vi "Teleop.vi"(10 "Match Info":T2={"Autonomous Elapsed Seconds"=0.0, "TeleOp Elapsed Seconds"=0.0, "Disabled Elapsed Seconds"=0.0, "Visited Autonomous"=FALSE, "Visited TeleOp"=FALSE, "Visited Disabled"=FALSE, "Autonomous Settings"={"Autonomous Style"=enum."Independent", "VI Refnum"=refnum}}, 11 "Call Context":T3) -> ()   [LabVIEW 2020]
doc: "This VI is called for each TeleOp packet received from the DS where the robot is not disabled. It is often used to read from the joysticks and update I/O or to update setpoints for timed control loops. It should complete and return within 20 milliseconds or it may miss DS packets."
uses:
  <vilib>/Rock Robotics/WPI/DriverStation/WPI_DriverStationDerivedRobotMode.ctl
  <vilib>/Rock Robotics/WPI/DriverStation/WPI_DriverStationMatch Info.ctl
  <vilib>/Rock Robotics/WPI/ThirdParty/Phoenix-LabVIEW/Motor Controller/Controls/CTRE_Phoenix_MotorControl_ControlMode.ctl
  <vilib>/Rock Robotics/WPI/ThirdParty/Phoenix-LabVIEW/CANCoder/Get/CTRE_Phoenix_CANcoder_GetSensorData.vi
  <vilib>/Rock Robotics/WPI/ThirdParty/Phoenix-LabVIEW/Pigeon IMU/CTRE_PigeonIMU_GetYPR.vi
panel:
  in  "FR PID gains":T1={"proportional gain (Kc)"=0.01, "integral time (Ti, min)"=0.0, "derivative time (Td, min)"=0.0} {"derivative time (Td, min)" format="%.3f"; "integral time (Ti, min)" format="%.3f"; "proportional gain (Kc)" format="%.6f"}
  in  "FL PID gains":T1={"proportional gain (Kc)"=0.01, "integral time (Ti, min)"=0.0, "derivative time (Td, min)"=0.0} {"derivative time (Td, min)" format="%.3f"; "integral time (Ti, min)" format="%.3f"; "proportional gain (Kc)" format="%.6f"}
  in  "BR PID gains":T1={"proportional gain (Kc)"=0.01, "integral time (Ti, min)"=0.0, "derivative time (Td, min)"=0.0} {"derivative time (Td, min)" format="%.3f"; "integral time (Ti, min)" format="%.3f"; "proportional gain (Kc)" format="%.6f"}
  in  "BL PID gains":T1={"proportional gain (Kc)"=0.01, "integral time (Ti, min)"=0.0, "derivative time (Td, min)"=0.0} {"derivative time (Td, min)" format="%.3f"; "integral time (Ti, min)" format="%.3f"; "proportional gain (Kc)" format="%.6f"}
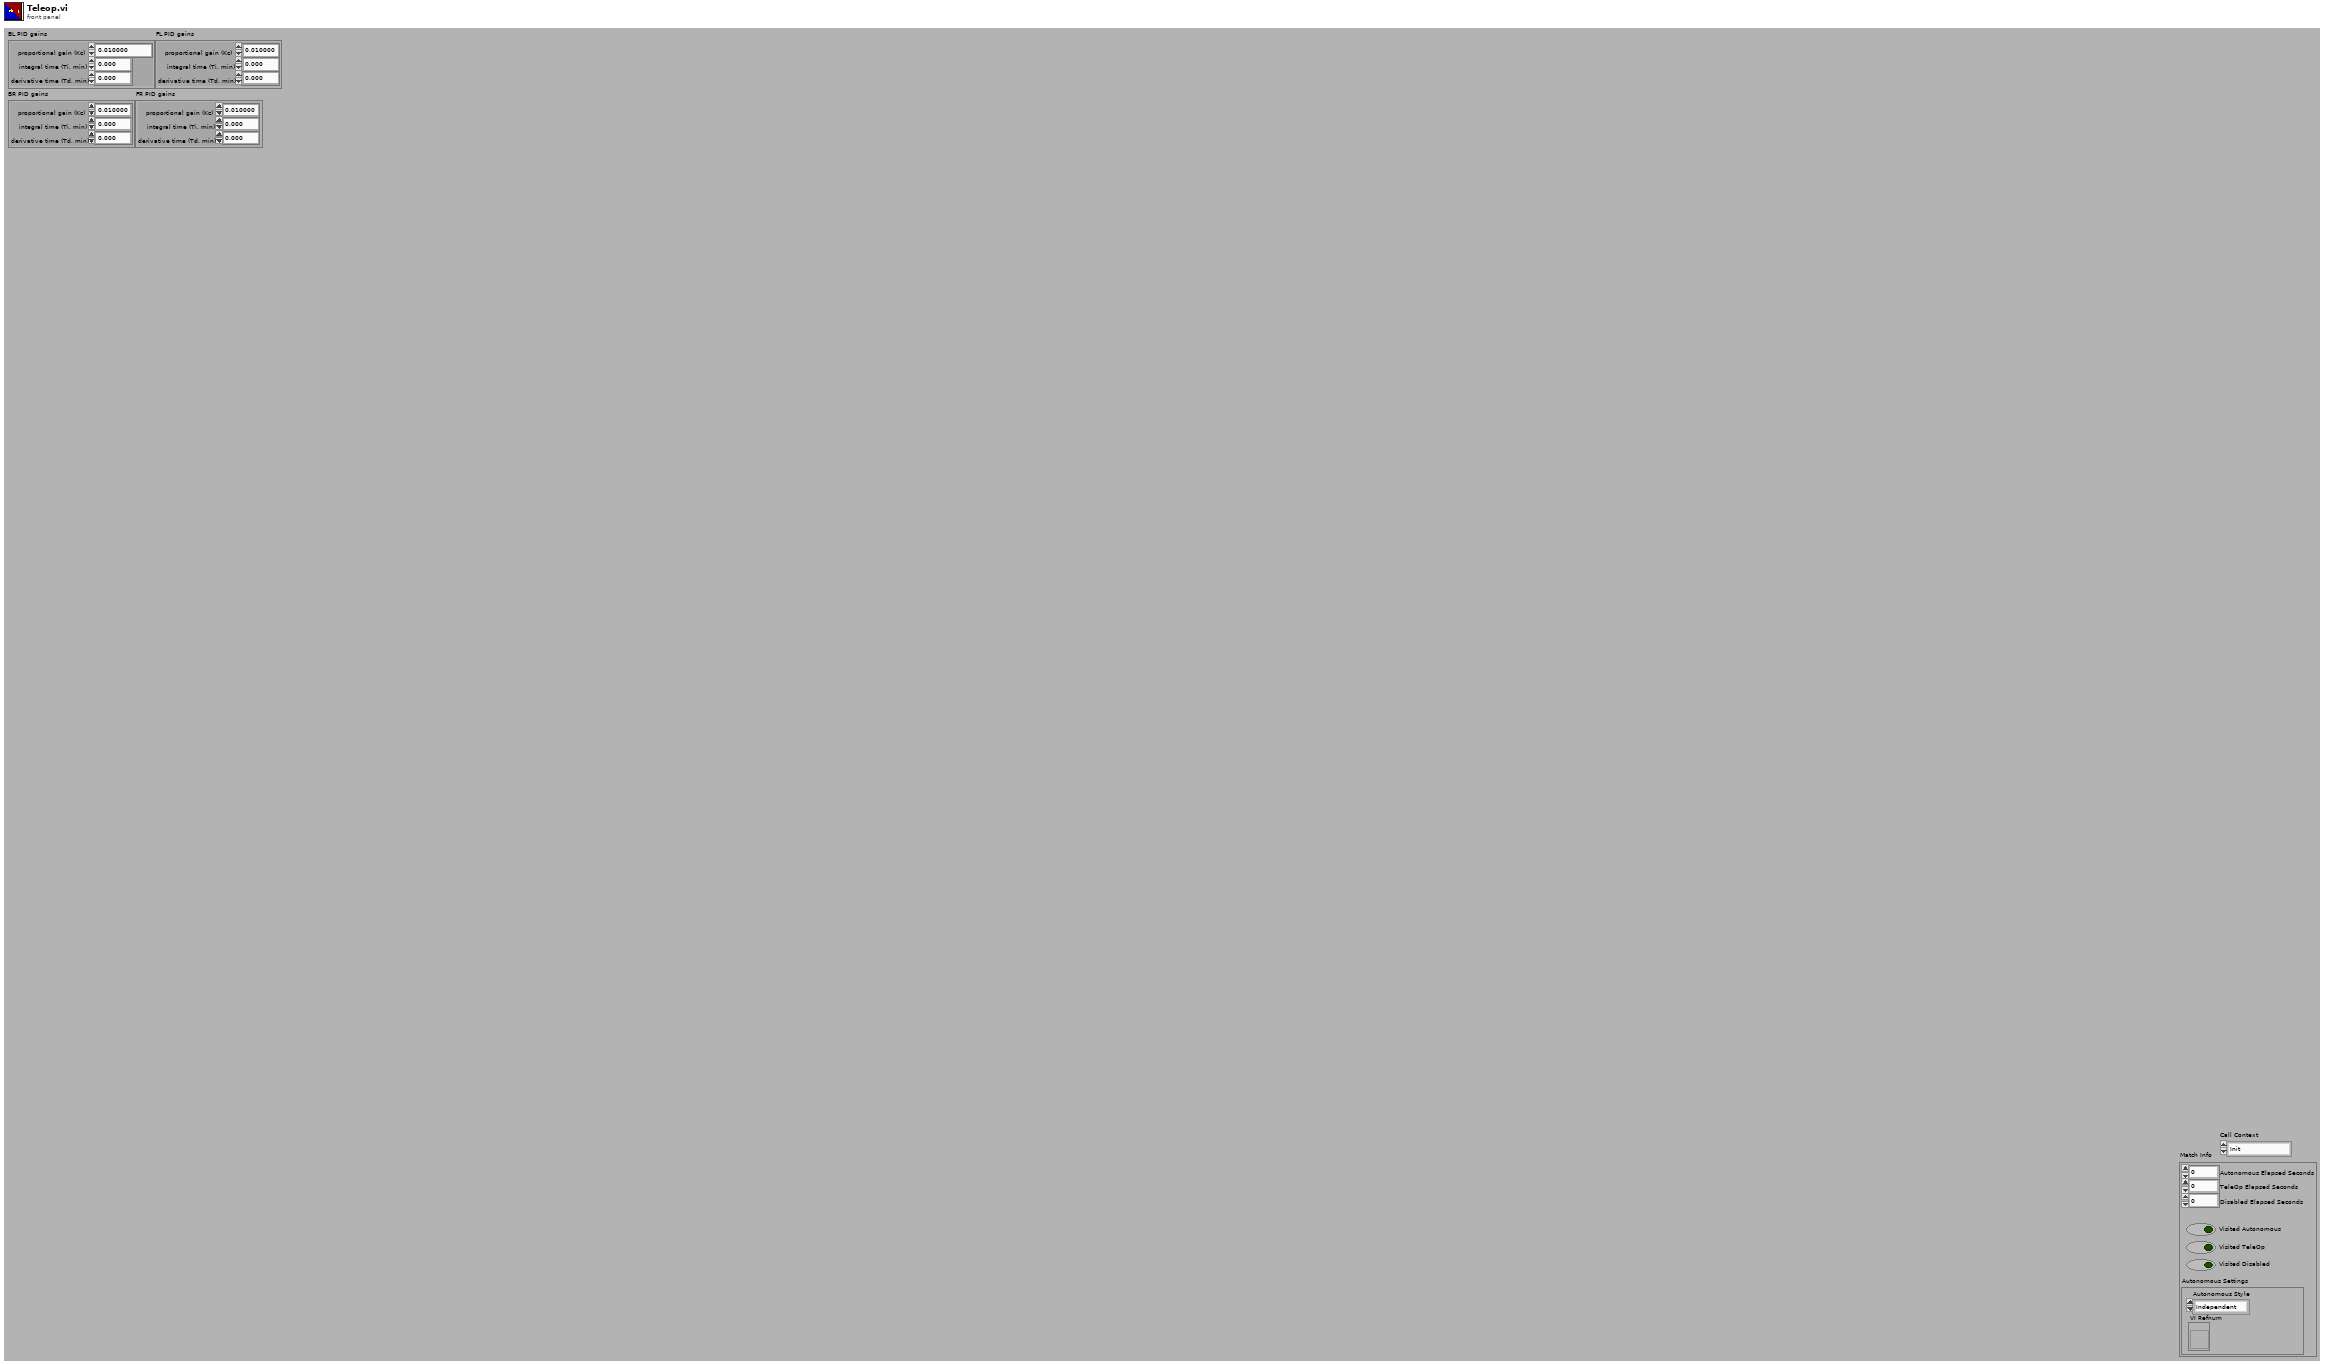
[diagram p1: front panel]
types:
  T1 = cluster{"proportional gain (Kc)":dbl, "integral time (Ti, min)":dbl, "derivative time (Td, min)":dbl}
  T2 = typedef "WPI_DriverStationMatch Info.ctl" = cluster{"Autonomous Elapsed Seconds":dbl, "TeleOp Elapsed Seconds":dbl, "Disabled Elapsed Seconds":dbl, "Visited Autonomous":bool, "Visited TeleOp":bool, "Visited Disabled":bool, "Autonomous Settings":cluster{"Autonomous Style":enum16{"Iterative", "Independent"}, "VI Refnum":refnum<vi>}}
  T3 = typedef "WPI_DriverStationDerivedRobotMode.ctl" = enum16{"Init", "Execute", "Stop"}
  T4 = typedef "CTRE_Phoenix_MotorControl_ControlMode.ctl" = u16
  T5 = cluster{"A":bool, "B":bool, "X":bool, "Y":bool, "Left Bumper":bool, "Right Bumper":bool, "View Button":bool, "Menu Button":bool, "Left Joystick Press":bool, "Right Joystick Press":bool, "Left Thumbpad X Axis":dbl, "Left Thumbpad Y Axis":dbl, "Left Trigger":dbl, "Right Trigger":dbl, "Right Thumbpad X Axis":dbl, "Right Thumbpad Y Axis":dbl, "Driver - Trigger":bool, "Driver - Middle Thumb":bool, "Driver - Left Thumb":bool, "Driver - Right Thumb":bool, "Driver - Left Top Left ":bool, "Driver - Left Top Middle":bool, "Driver - Left Top Right":bool, "Driver - Left Bottom Right":bool, "Driver - Left Bottom Middle":bool, "Driver - Left Bottom Left":bool, "Driver - Right Top Right":bool, "Driver - Right Top Middle":bool, "Driver - Right Top Left":bool, "Driver - Right Bottom Left":bool, "Driver - Right Bottom Middle":bool, "Driver - Right Bottom Right":bool, "Driver - X Axis":dbl, "Driver - Y Axis":dbl, "Driver - Z Axis":dbl}
  T6 = typedef "CTRE_PigeonIMU_DeviceRef.ctl" = cluster{"DeviceStatus":errorcluster, "Device Number":u8, "Type":T7, "Device ID":u32, "Handle":u64, "UsageFrame":u32, "Library Path":path}
  T7 = typedef "CTRE_PigeonIMU_ConnectionType.ctl" = u32
  T8 = typedef "CTRE_Phoenix_CANcoder_DeviceRef.ctl" = cluster{"DeviceStatus":errorcluster, "Device Number":u8, "Handle":u64, "UsageFrame":u32, "Library Path":path}
  T9 = typedef "WPI_MotorControlDeviceRef.ctl" = cluster{"DeviceStatus":errorcluster, "Type":T10, "PWM":cluster{"PWM Channel":T11, "DeadBand":T12}, "CAN":cluster{"Device Number":u8, "SetOutput VI Ref":variant, "GetOutput VI Ref":variant, "Enable VI Ref":variant, "Disable VI Ref":variant, "Data":variant}, "Invert":bool, "DIO PWM":cluster{"PWM \"Enable\" Channel":T11, "DIOChannel":T13, "PWM Rate":dbl}}
  T10 = typedef "WPI_MotorControlType.ctl" = enum16{"PWM", "CAN", "DIO PWM"}
  T11 = typedef "FPGA_DIOPWMChannel.ctl" = enum8{"PWM 0", "PWM 1", "PWM 2", "PWM 3", "PWM 4", "PWM 5", "PWM 6", "PWM 7", "PWM 8", "PWM 9", "PWM MXP 0", "PWM MXP 1", "PWM MXP 2", "PWM MXP 3", "PWM MXP 4", "PWM MXP 5", "PWM MXP 6", "PWM MXP 7", "PWM MXP 8", "PWM MXP 9", "Invalid"}
  T12 = typedef "WPI_PWMDeadband.ctl" = cluster{"Name":string, "maxPositivePwm":i32, "minPositivePwm":i32, "centerPwm":i32, "maxNegativePwm":i32, "minNegativePwm":i32, "angularRange":u16}
  T13 = typedef "FPGA_DIOChannel.ctl" = enum8{"DIO 0", "DIO 1", "DIO 2", "DIO 3", "DIO 4", "DIO 5", "DIO 6", "DIO 7", "DIO 8", "DIO 9", "DIO MXP 0", "DIO MXP 1", "DIO MXP 2", "DIO MXP 3", "DIO MXP 4", "DIO MXP 5", "DIO MXP 6", "DIO MXP 7", "DIO MXP 8", "DIO MXP 9", "DIO MXP 10", "DIO MXP 11", "DIO MXP 12", "DIO MXP 13", "DIO MXP 14", "DIO MXP 15", "SPI Port CS1", "SPI Port CS2", "SPI Port CS3", "SPI Port MISO", "SPI Port MOSI", "Invalid"}
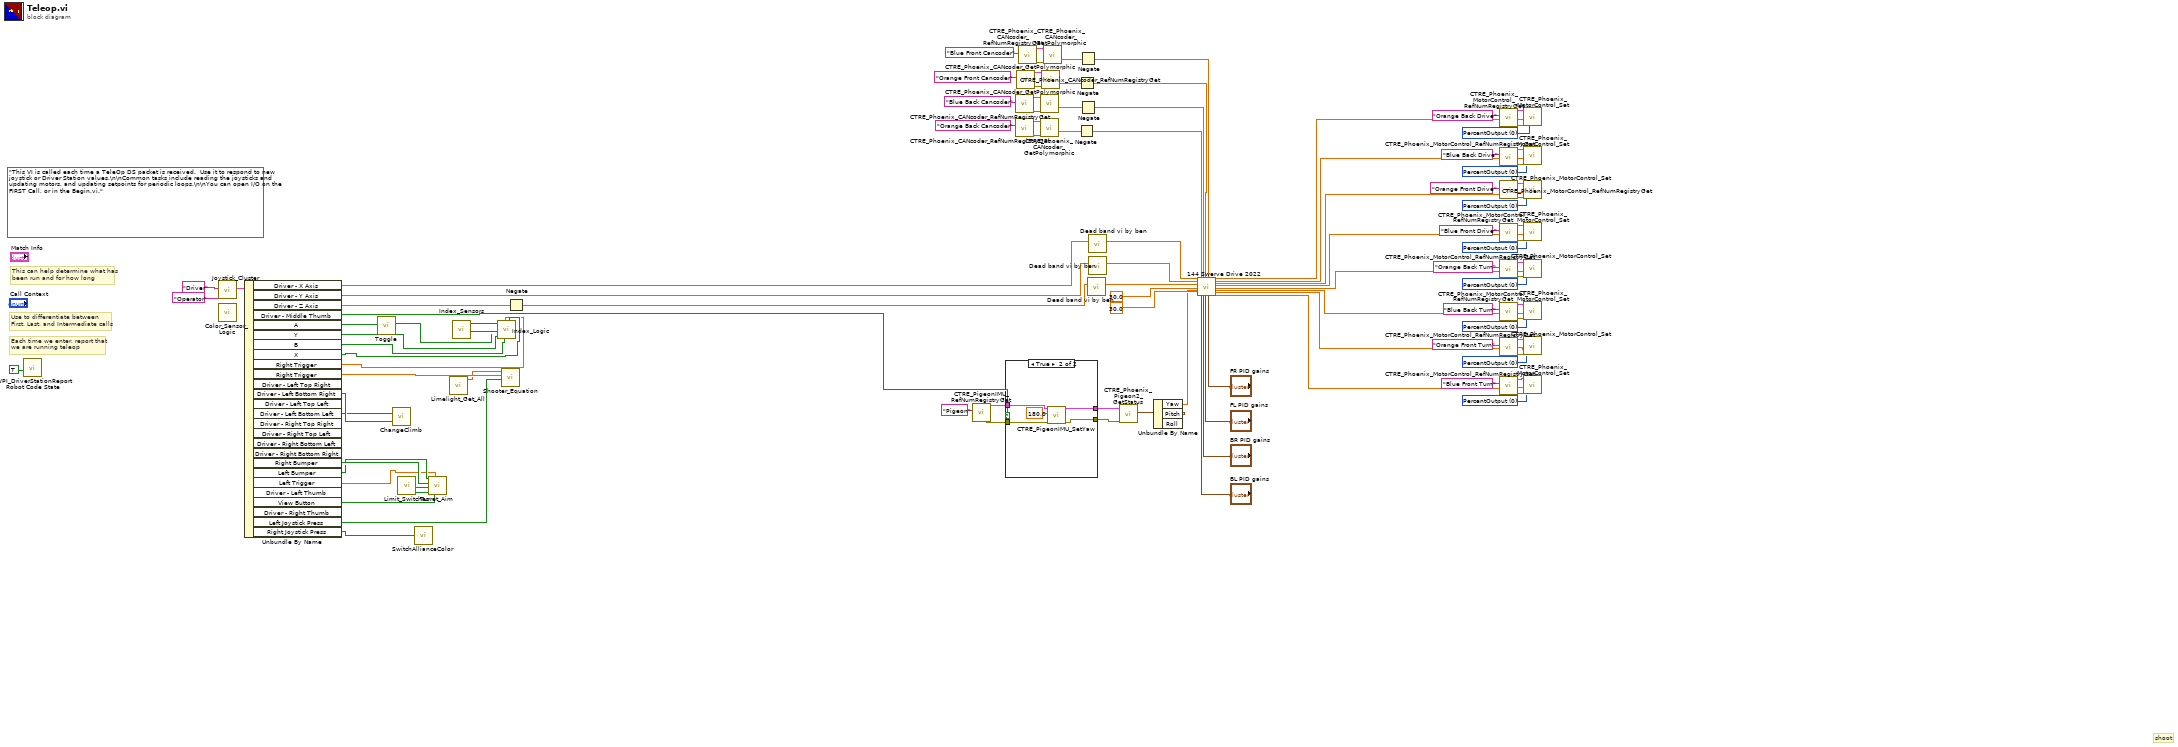
[diagram p0: block diagram]
diagram:
  w21 = T4 0 items=["PercentOutput"=0, "Position"=1, "Velocity"=2, "Current"=3, "Follower"=5, "MotionProfile"=6, "MotionMagic"=7, "MotionProfileArc"=10, "Disabled"=15] ("Control Mode")
  w25 = T4 0 items=["PercentOutput"=0, "Position"=1, "Velocity"=2, "Current"=3, "Follower"=5, "MotionProfile"=6, "MotionMagic"=7, "MotionProfileArc"=10, "Disabled"=15] ("Control Mode")
  w28 = T4 0 items=["PercentOutput"=0, "Position"=1, "Velocity"=2, "Current"=3, "Follower"=5, "MotionProfile"=6, "MotionMagic"=7, "MotionProfileArc"=10, "Disabled"=15] ("Control Mode")
  w32 = T4 0 items=["PercentOutput"=0, "Position"=1, "Velocity"=2, "Current"=3, "Follower"=5, "MotionProfile"=6, "MotionMagic"=7, "MotionProfileArc"=10, "Disabled"=15] ("Control Mode")
  w60 = T4 0 items=["PercentOutput"=0, "Position"=1, "Velocity"=2, "Current"=3, "Follower"=5, "MotionProfile"=6, "MotionMagic"=7, "MotionProfileArc"=10, "Disabled"=15] ("Control Mode")
  w64 = T4 0 items=["PercentOutput"=0, "Position"=1, "Velocity"=2, "Current"=3, "Follower"=5, "MotionProfile"=6, "MotionMagic"=7, "MotionProfileArc"=10, "Disabled"=15] ("Control Mode")
  w67 = T4 0 items=["PercentOutput"=0, "Position"=1, "Velocity"=2, "Current"=3, "Follower"=5, "MotionProfile"=6, "MotionMagic"=7, "MotionProfileArc"=10, "Disabled"=15] ("Control Mode")
  w11 = T4 0 items=["PercentOutput"=0, "Position"=1, "Velocity"=2, "Current"=3, "Follower"=5, "MotionProfile"=6, "MotionMagic"=7, "MotionProfileArc"=10, "Disabled"=15] ("Control Mode")
  (unwired) "This VI is called each time a TeleOp DS packet is received.  Use it to respond to new joystick or Driver Station values.\n\nCommon tasks include reading the joysticks and updating motors, and updating setpoints for periodic loops.\n\nYou can open I/O on the FIRST Call, or in the Begin.vi."
  # "shoot"
  # "Each time we enter, report that\nwe are running teleop"
  # "Use to differentiate between\nFirst, Last, and Intermediate calls"
  # "This can help determine what has\nbeen run and for how long"
  n1 = call <vilib>:"WPI_DriverStationReport Robot Code State.vi"("TeleOp"=TRUE ("Autonomous")) -> ()  [unwired: 10 in, 1 out]
  n2 = call "Joystick_Cluster.vi"("Xbox"="Operator", "Thrustmaster"="Driver") -> ("Joystick Output"=w102:T5)  [unwired: 9 in]
  n3 = call "Color_Sensor_Logic.vi"() -> ()  [unwired: 12 in]
  n4 = Unbundle By Name(w102) -> ("Driver - X Axis"=w43:dbl, "Driver - Y Axis"=w42:dbl, "Driver - Z Axis"=w41:dbl, "Driver - Middle Thumb"=w48:bool, "A"=w97:bool, "Y"=w99:bool, "B"=w98:bool, "X"=w9:bool, "Right Trigger"=w5:dbl, "Right Trigger"=w3:dbl, "Driver - Left Bottom Right"=w8:bool, "Driver - Left Bottom Left"=w7:bool, "Right Bumper"=w93:bool, "Left Bumper"=w92:bool, "Left Trigger"=w91:dbl, "View Button"=w90:bool, "Left Joystick Press"=w4:bool, "Right Joystick Press"=w6:bool)  [unwired: 8 out]
  n5 = call "Toggle.vi"("Boolean"=w97) -> ("Boolean Out"=w96:bool)
  n6 = call "ChangeClimb.vi"("Mid"=w8, "Low"=w7) -> ()  [unwired: 1 in]
  n7 = call "Limit_Switches.vi"() -> ("Blue Limit Pressed"=w94:bool, "Orange Limit Pressed"=w95:bool)  [unwired: 10 in]
  n8 = call "SwitchAllianceColor.vi"("Pressed"=w6) -> ()  [unwired: 1 in]
  n9 = call "Turret_Aim.vi"("View Button"=w90, "Left Trigger"=w91, "Orange Limit Pressed"=w95, "Blue Limit Pressed"=w94, "Right Bumper"=w93, "Left Bumper"=w92) -> ()  [unwired: 6 in]
  n10 = call "Limelight_Get_All.vi"() -> ("Ty"=w2:dbl)  [unwired: 10 in, 1 out]
  n11 = call "Index_Sensors.vi"() -> ("Intake Pressed"=w101:bool, "Elevate Pressed"=w100:bool)  [unwired: 9 in, 1 out]
  n12 = call "Index_Logic.vi"("Intake Pressed"=w101, "X"=w9, "B"=w98, "Right Trigger"=w5, "Y"=w99, "A"=w96, "Elevate Pressed"=w100) -> ()  [unwired: 5 in]
  n13 = call "Shooter_Equation.vi"("Left Bumper"=w4, "Right Trigger"=w3, "Ty"=w2) -> ()  [unwired: 9 in]
  n14 = Negate(x=w41) -> (-x=w1:dbl)
  n15 = call <vilib>:"CTRE_PigeonIMU_RefNumRegistryGet.vi"("refnum name"="Pigeon") -> ("error out"=w57:errorcluster, "PigeonIMUDevRef"=w58:T6)  [unwired: 9 in]
  n16 = case shown="True" w48 {
    tunnel: w58 -> [w107 w111]
    tunnel: w57 -> [w106 w110]
    tunnel: [w106 w109] -> w56
    tunnel: [w107 w108] -> w55
    frame False {
    }
    frame True {
      n17 = call <vilib>:"CTRE_PigeonIMU_SetYaw.vi"("error in (no error)"=w110, "Value"=180.0, "PigeonIMUDevRef"=w111) -> ("error out"=w109:errorcluster, "PigeonIMUDevRef"=w108:T6)  [unwired: 7 in]
    }
  }
  n18 = call <vilib>:"CTRE_Phoenix_CANcoder_RefNumRegistryGet.vi"("refnum name"="Blue Back Cancoder") -> ("error out"=w84:errorcluster, "CTRE_CANcoder_DeviceRef"=w85:T8)  [unwired: 9 in]
  n19 = call <vilib>:"CTRE_Phoenix_CANcoder_RefNumRegistryGet.vi"("refnum name"="Orange Back Cancoder") -> ("error out"=w86:errorcluster, "CTRE_CANcoder_DeviceRef"=w87:T8)  [unwired: 9 in]
  n20 = call <vilib>:"CTRE_Phoenix_CANcoder_RefNumRegistryGet.vi"("refnum name"="Orange Front Cancoder") -> ("error out"=w88:errorcluster, "CTRE_CANcoder_DeviceRef"=w89:T8)  [unwired: 9 in]
  n21 = call <vilib>:"CTRE_Phoenix_CANcoder_RefNumRegistryGet.vi"("refnum name"="Blue Front Cancoder") -> ("error out"=w82:errorcluster, "CTRE_CANcoder_DeviceRef"=w83:T8)  [unwired: 9 in]
  n22 = call-poly <vilib>:"CTRE_Phoenix_CANcoder_GetPolymorphic.vi"("CTRE_CANcoder_DeviceRef"=w85, "error in"=w84) -> ("Absolute Position"=w77:dbl)  [unwired: 9 in, 4 out]
  n23 = call-poly <vilib>:"CTRE_Phoenix_CANcoder_GetPolymorphic.vi"("CTRE_CANcoder_DeviceRef"=w87, "error in"=w86) -> ("Absolute Position"=w75:dbl)  [unwired: 9 in, 4 out]
  n24 = call-poly <vilib>:"CTRE_Phoenix_CANcoder_GetPolymorphic.vi"("CTRE_CANcoder_DeviceRef"=w89, "error in"=w88) -> ("Absolute Position"=w74:dbl)  [unwired: 9 in, 4 out]
  n25 = call-poly <vilib>:"CTRE_Phoenix_CANcoder_GetPolymorphic.vi"("CTRE_CANcoder_DeviceRef"=w83, "error in"=w82) -> ("Absolute Position"=w76:dbl)  [unwired: 9 in, 4 out]
  n26 = Negate(x=w75) -> (-x=w47:dbl)
  n27 = Negate(x=w74) -> (-x=w45:dbl)
  n28 = Negate(x=w76) -> (-x=w44:dbl)
  n29 = Negate(x=w77) -> (-x=w46:dbl)
  n30 = call "Dead band vi by ben.vi"("Numeric"=w1) -> ("Deadbanded Value"=w38:dbl)  [unwired: 10 in]
  n31 = call "Dead band vi by ben.vi"("Numeric"=w43) -> ("Deadbanded Value"=w40:dbl)  [unwired: 10 in]
  n32 = call "Dead band vi by ben.vi"("Numeric"=w42) -> ("Deadbanded Value"=w39:dbl)  [unwired: 10 in]
  n33 = call-poly <vilib>:"CTRE_Phoenix_Pigeon2_GetStatus.vi"("error in (no error)"=w56, "PigeonIMUDevRef"=w55) -> ("Yaw Pitch Roll"=w53:cluster{"Yaw":dbl, "Pitch":dbl, "Roll":dbl})  [unwired: 7 in, 2 out]
  n34 = Unbundle By Name(w53) -> ("Yaw"=w10:dbl)  [unwired: 2 out]
  n35 = call "144 Swerve Drive 2022.vi"("Joystick X"=w40, "Joystick Y"=w39, "Joystick Z"=w38, "Robot Length(in.)"=30.0, "Robot Width(in.)"=30.0, "Gyro"=w10, "BL_Steer_Encoder"=w47, "BL PID gains"="BL PID gains", "BR_Steer_Encoder"=w46, "BR PID gains"="BR PID gains", "FL_Steer_Encoder"=w45, "FL PID gains"="FL PID gains", "FR_Steer_Encoder"=w44, "FR PID gains"="FR PID gains") -> ("Throttle BL"=w19:dbl, "Throttle BR"=w18:dbl, "Throttle FL"=w17:dbl, "Throttle FR"=w16:dbl, "BL_STEER_MOTOR_OUTPUT"=w15:dbl, "BR_STEER_MOTOR_OUTPUT"=w14:dbl, "FL_STEER_MOTOR_OUTPUT"=w13:dbl, "FR_STEER_MOTOR_OUTPUT"=w12:dbl)  [unwired: 6 in]
  n36 = call <vilib>:"CTRE_Phoenix_MotorControl_RefNumRegistryGet.vi"("refnum name"="Orange Back Drive") -> ("error out"=w72:errorcluster, "PhoenixMotorControlDevRef"=w73:T9)  [unwired: 9 in]
  n37 = call <vilib>:"CTRE_Phoenix_MotorControl_RefNumRegistryGet.vi"("refnum name"="Blue Back Drive") -> ("error out"=w69:errorcluster, "PhoenixMotorControlDevRef"=w70:T9)  [unwired: 9 in]
  n38 = call <vilib>:"CTRE_Phoenix_MotorControl_RefNumRegistryGet.vi"("refnum name"="Orange Front Drive") -> ("error out"=w66:errorcluster, "PhoenixMotorControlDevRef"=w63:T9)  [unwired: 9 in]
  n39 = call <vilib>:"CTRE_Phoenix_MotorControl_RefNumRegistryGet.vi"("refnum name"="Blue Front Drive") -> ("error out"=w62:errorcluster, "PhoenixMotorControlDevRef"=w59:T9)  [unwired: 9 in]
  n40 = call <vilib>:"CTRE_Phoenix_MotorControl_RefNumRegistryGet.vi"("refnum name"="Orange Back Turn") -> ("error out"=w34:errorcluster, "PhoenixMotorControlDevRef"=w35:T9)  [unwired: 9 in]
  n41 = call <vilib>:"CTRE_Phoenix_MotorControl_RefNumRegistryGet.vi"("refnum name"="Blue Back Turn") -> ("error out"=w30:errorcluster, "PhoenixMotorControlDevRef"=w31:T9)  [unwired: 9 in]
  n42 = call <vilib>:"CTRE_Phoenix_MotorControl_RefNumRegistryGet.vi"("refnum name"="Orange Front Turn") -> ("error out"=w27:errorcluster, "PhoenixMotorControlDevRef"=w24:T9)  [unwired: 9 in]
  n43 = call <vilib>:"CTRE_Phoenix_MotorControl_RefNumRegistryGet.vi"("refnum name"="Blue Front Turn") -> ("error out"=w23:errorcluster, "PhoenixMotorControlDevRef"=w20:T9)  [unwired: 9 in]
  n44 = call <vilib>:"CTRE_Phoenix_MotorControl_Set.vi"("error in (no error)"=w72, "Output"=w19, "Control Mode"=w11, "PhoenixMotorControlDevRef"=w73) -> ()  [unwired: 6 in, 2 out]
  n45 = call <vilib>:"CTRE_Phoenix_MotorControl_Set.vi"("error in (no error)"=w69, "Output"=w18, "Control Mode"=w67, "PhoenixMotorControlDevRef"=w70) -> ()  [unwired: 6 in, 2 out]
  n46 = call <vilib>:"CTRE_Phoenix_MotorControl_Set.vi"("error in (no error)"=w66, "Output"=w17, "Control Mode"=w64, "PhoenixMotorControlDevRef"=w63) -> ()  [unwired: 6 in, 2 out]
  n47 = call <vilib>:"CTRE_Phoenix_MotorControl_Set.vi"("error in (no error)"=w62, "Output"=w16, "Control Mode"=w60, "PhoenixMotorControlDevRef"=w59) -> ()  [unwired: 6 in, 2 out]
  n48 = call <vilib>:"CTRE_Phoenix_MotorControl_Set.vi"("error in (no error)"=w34, "Output"=w15, "Control Mode"=w32, "PhoenixMotorControlDevRef"=w35) -> ()  [unwired: 6 in, 2 out]
  n49 = call <vilib>:"CTRE_Phoenix_MotorControl_Set.vi"("error in (no error)"=w30, "Output"=w14, "Control Mode"=w28, "PhoenixMotorControlDevRef"=w31) -> ()  [unwired: 6 in, 2 out]
  n50 = call <vilib>:"CTRE_Phoenix_MotorControl_Set.vi"("error in (no error)"=w27, "Output"=w13, "Control Mode"=w25, "PhoenixMotorControlDevRef"=w24) -> ()  [unwired: 6 in, 2 out]
  n51 = call <vilib>:"CTRE_Phoenix_MotorControl_Set.vi"("error in (no error)"=w23, "Output"=w12, "Control Mode"=w21, "PhoenixMotorControlDevRef"=w20) -> ()  [unwired: 6 in, 2 out]
